vi "read.vi"(4 "Gain":refnum<vi>, 5 "Exposure":refnum<vi>, 6 "Actual Rate":refnum<vi>, 7 "Video Display":refnum<vi>, 8 "error in":errorcluster, 9 "Stop Flag Reference":refnum<vi>, 10 "VISA resource name":refnum<visa-resource-name>, 11 "Imaging in":refnum<class "Imaging.lvclass">) -> (0 "error out":errorcluster, 3 "Imaging out":refnum<class "Imaging.lvclass">)   [LabVIEW 2014, in "Imaging.lvclass"]
uses:
  Imaging.lvclass
  <vilib>/vision/driver/IMAQdx.llb/IMAQdx Buffer Number Mode.ctl
  <vilib>/vision/driver/NI_Vision_Acquisition_Software.lvlib
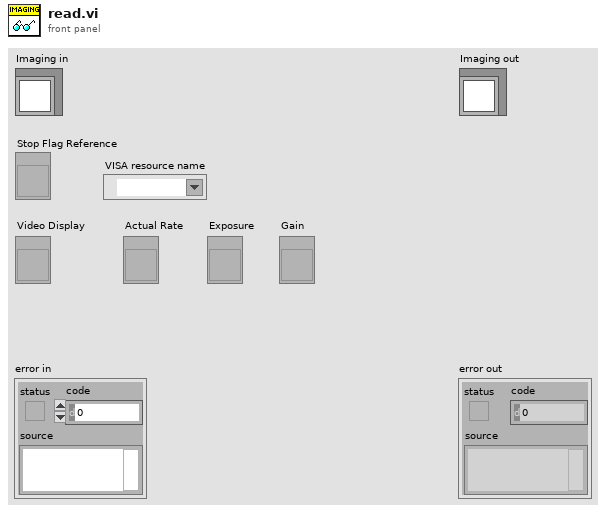
[diagram p1: front panel]
types:
  T1 = typedef "IMAQdx.ctl" = refnum<k21>
  T2 = typedef "IMAQ Image.ctl" = refnum<image>
  T3 = typedef "NI_Vision_Acquisition_Software.lvlib/IMAQdx Buffer Number Mode.ctl" = enum32{"Next", "Last", "Buffer Number", "Every", "Last New"}
  T4 = cluster{"Image Out":T2, dbl, "seconds since 1Jan1904":timestamp}
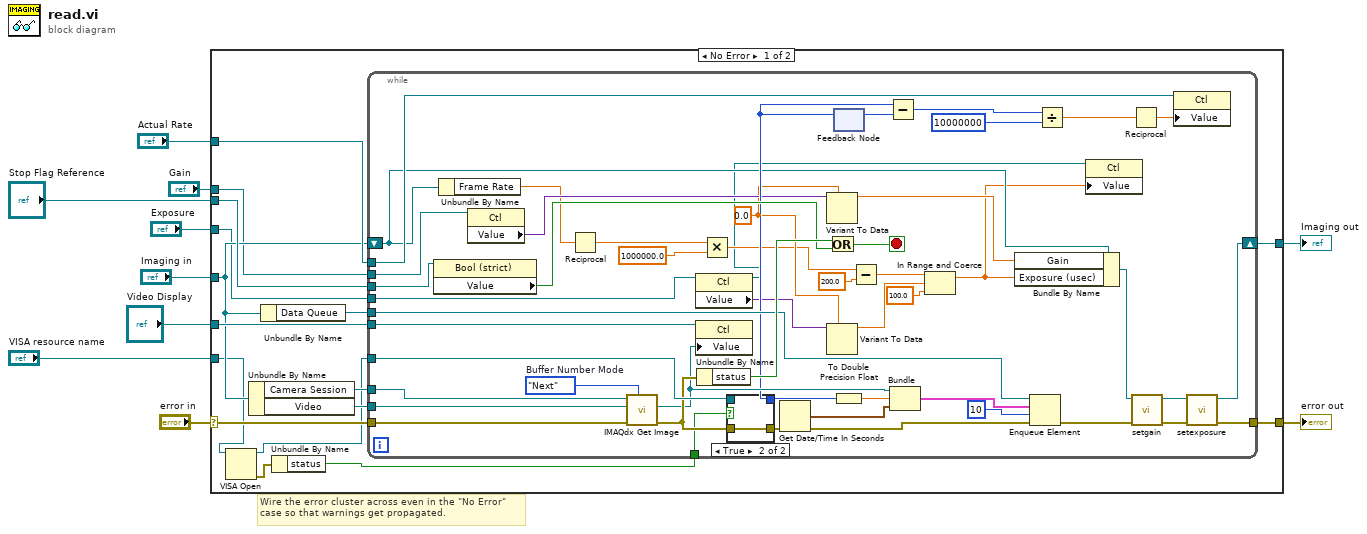
[diagram p0: block diagram]
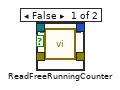
[diagram p2: hidden frame]
diagram:
  # "Wire the error cluster across even in the \"No Error\"\ncase so that warnings get propagated."
  n1 = case shown="No Error" "error in" {
    selector: "error in" -> [w24 w82]
    tunnel: [w23 w82] -> w9
    tunnel: [w17 w81] -> w7
    tunnel: "Imaging in" -> [w18 w81]
    tunnel: "Stop Flag Reference" -> [w26 _]
    tunnel: "VISA resource name" -> [w12 _]
    tunnel: "Video Display" -> [w20 _]
    tunnel: "Actual Rate" -> [w19 _]
    tunnel: "Gain" -> [w16 _]
    tunnel: "Exposure" -> [w15 _]
    frame No Error {
      n2 = VISA Open(VISA resource name=w12) -> (VISA resource name=w11:refnum<visa-resource-name>, error out=w14:errorcluster)  [unwired: 4 in]
      n3 = Unbundle By Name(w18) -> ("Camera Session"=w22:T1, "Video"=w21:T2)
      n4 = Unbundle By Name(w18) -> ("Data Queue"=w25:refnum<queue>)
      n5 = Unbundle By Name(w14) -> ("status"=w13:bool)
      n6 = while {
        tunnel: w24 -> [w72]
        tunnel: w22 -> [w73]
        tunnel: w21 -> [w71]
        tunnel: w25 -> [w67]
        tunnel: w26 -> [w65]
        tunnel: w11 -> [w63]
        tunnel: [w41] -> w23
        tunnel: w20 -> [w60]
        tunnel: w19 -> [w53]
        shift-right: [w44] -> w17
        shift-left: w18 -> [w37]
        tunnel: w16 -> [w51]
        tunnel: w15 -> [w50]
        tunnel: w13 -> [w27]
        stop <- w75 stop-if-true
        w47 = 0.0
        w70 = IMAQdx_Buffer_Number_Mode."Next"  # Buffer Number Mode
        n7 = property class="Bool (strict)"(reference=w65) -> ("Value"=w64:bool)  [unwired: 1 in, 2 out]
        n8 = Unbundle By Name(w37) -> ("Frame Rate"=w36:dbl)
        n9 = property class="Ctl"(reference=w51) -> ("Value"=w48:variant)  [unwired: 1 in, 2 out]
        n10 = Reciprocal(x=w36) -> (1/x=w35:dbl)
        n11 = call <vilib>:"IMAQdx Get Image.vi"("Buffer Number Mode (Next)"=w70, "error in"=w72, "Image In"=w71, "Session In"=w73) -> ("error out"=w62:errorcluster, "Image Out"=w59:T2)  [unwired: 1 in, 5 out]
        n12 = property class="Ctl"(reference=w50) -> (reference out=w30:refnum<vi>, "Value"=w49:variant)  [unwired: 1 in, 1 out]
        n13 = property class="Ctl"(reference=w60, "Value"=w59) -> ()  [unwired: 1 in, 2 out]
        n14 = Unbundle By Name(w62) -> ("status"=w74:bool)
        n15 = Multiply(x=w35, y=1000000.0) -> (x*y=w32:dbl)
        n16 = case shown="True" w27 {
          tunnel: w63 -> [w79 _]
          tunnel: w62 -> [w78 w80]
          tunnel: [w77 w80] -> w61
          tunnel: [w76 _] -> w57
          frame False {
            n17 = call "ReadFreeRunningCounter.vi"("error in"=w78, "VISA resource name"=w79) -> ("error out"=w77:errorcluster, "Counter Data"=w76:u32)  [unwired: 8 in]
          }
          frame True {
          }
        }
        n18 = Get Date/Time In Seconds() -> (seconds since 1Jan1904=w28:timestamp)
        n19 = Variant To Data(type=w47, Variant=w48) -> (data=w38:dbl)  [unwired: 1 in, 1 out]
        n20 = Variant To Data(type=w47, Variant=w49) -> (data=w40:dbl)  [unwired: 1 in, 1 out]
        n21 = Or(x=w74, y=w64) -> (x .or. y?=w75:bool)
        n22 = feedback-in #1(w57) -> ()
        n23 = feedback #1() -> (w58:u32)  [unwired: 1 in]
        n24 = To Double Precision Float(number=w57) -> (double precision float=w66:dbl)
        n25 = Subtract(x=w32, y=200.0) -> (x-y=w33:dbl)
        n26 = Subtract(x=w57, y=w58) -> (x-y=w56:u32)
        n27 = Bundle("Image Out"=w59, w66, "seconds since 1Jan1904"=w28) -> (w68:T4)  [unwired: 1 in]
        n28 = In Range and Coerce(upper limit=w33, x=w40, lower limit=100.0) -> (coerced(x)=w29:dbl)  [unwired: 1 out]
        n29 = Bundle By Name(cluster=w37, "Gain"=w38, "Exposure (usec)"=w29) -> (w46:refnum<class "Imaging.lvclass">)
        n30 = Enqueue Element(queue=w67, element=w68, timeout in ms (-1)=10, error in (no error)=w61) -> (error out=w43:errorcluster)  [unwired: 2 out]
        n31 = Divide(x=w56, y=u32 10000000) -> (x/y=w54:dbl)
        n32 = property class="Ctl"(reference=w30, "Value"=w29) -> ()  [unwired: 1 in, 2 out]
        n33 = Reciprocal(x=w54) -> (1/x=w52:dbl)
        n34 = call-dynamic "setgain.vi"("error in (no error)"=w43, "Imaging in"=w46) -> ("error out"=w42:errorcluster, "Imaging out"=w45:refnum<class "Imaging.lvclass">)  [unwired: 8 in]
        n35 = property class="Ctl"(reference=w53, "Value"=w52) -> ()  [unwired: 1 in, 2 out]
        n36 = call-dynamic "setexposure.vi"("error in (no error)"=w42, "Imaging in"=w45) -> ("error out"=w41:errorcluster, "Imaging out"=w44:refnum<class "Imaging.lvclass">)  [unwired: 8 in]
      }
    }
    frame Error {
    }
  }
  "error out" <- w9
  "Imaging out" <- w7
